vi "Initialize Sessions.vi"   [LabVIEW 2020, in "MeasurementLink niDigital.lvlib"]
doc: "Create the NI-Digital driver session(s) from a reservation."
uses:
  MeasurementLink niDigital.lvlib
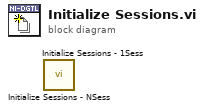
[diagram p0: block diagram]
diagram:
  n1 = call "Initialize Sessions - NSess.vi"() -> ()  [unwired: 8 in, 4 out]
  n2 = call "Initialize Sessions - 1Sess.vi"() -> ()  [unwired: 8 in, 4 out]
